vi "TranslationStage_UI_launcher.vi"   [LabVIEW 2023]
uses:
  <vilib>/ActorFramework/Actor/Actor.lvclass
  TranslationStage_UI/TranslationStageUI.lvclass
  C:/Program Files/National Instruments/LabVIEW 2023/vi.lib/ActorFramework/Actor/Actor.lvclass
  C:/Users/quantum/Documents/LVDAQ/UIs/TranslationStage_UI/TranslationStage_UI/TranslationStageUI.lvclass
  C:/Users/quantum/Documents/LVDAQ/Interfaces/InitDeinitInterface/InitDeinitComm/InitDeinitComm.lvclass
  C:/Users/quantum/Documents/LVDAQ/Interfaces/AbstractInstrumentClasses/TranslationStages_LV/TranslationStagesComm/TranslationStagesComm.lvclass
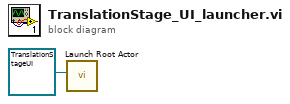
[diagram p0: block diagram]
diagram:
  n1 = call <vilib>:"Launch Root Actor.vi"("Actor"=refnum<class "TranslationStageUI.lvclass"> refnum ("TranslationStage_UI.lvlib:TranslationStageUI.lvclass")) -> ()  [unwired: 9 in, 2 out]
